vi "REPORT.Create line.vi"(7 "Secction":string, 10 "Char":string="-", 11 "Text In":string) -> (3 "Text Out":string)   [LabVIEW 2019]
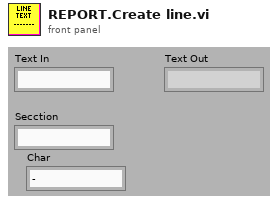
[diagram p1: front panel]
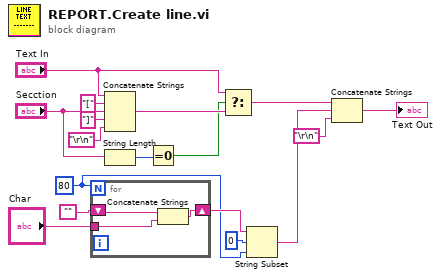
[diagram p0: block diagram]
diagram:
  w2 = 80
  n1 = for {
    N: w2 -> [_]
    shift-right: [w20] -> w4
    shift-left: "" -> [w19]
    tunnel: "Char" -> [w18]
    n2 = Concatenate Strings(w19, w18) -> (w20:string)
  }
  n3 = Concatenate Strings("Text In", "[" ("string"), "Secction", "]" ("string"), "\r\n") -> (w14:string)
  n4 = String Length(string="Secction") -> (length=w11:i32)
  n5 = Equal To 0?(x=w11) -> (x = 0?=w12:bool)
  n6 = Select(t="Text In", s=w12, f=w14) -> (s? t:f=w16:string)
  n7 = String Subset(string=w4, offset (0)=0, length (rest)=w2) -> (substring=w1:string)
  n8 = Concatenate Strings(w16, w1, "\r\n") -> (→"Text Out":string)
